vi "Wheel Angle (Ai).vi"(1 "Gamma ai":dbl, 2 "A":dbl) -> (0 "Ai":dbl)   [LabVIEW 2012]
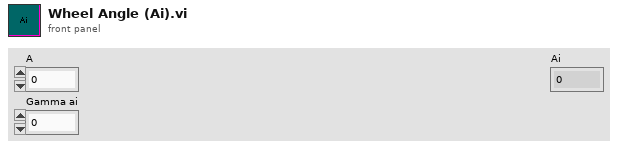
[diagram p1: front panel]
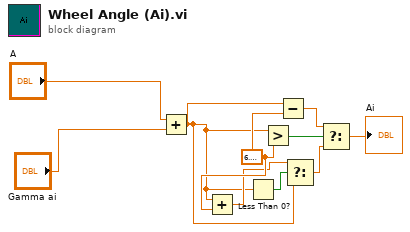
[diagram p0: block diagram]
diagram:
  w4 = 6.283185307179586
  n1 = Add(x="A", y="Gamma ai") -> (x+y=w2:dbl)
  n2 = Add(x=w2, y=w4) -> (x+y=w3:dbl)
  n3 = Less Than 0?(x=w2) -> (x < 0?=w5:bool)
  n4 = Greater?(x=w2, y=w4) -> (0:w8:bool)
  n5 = Subtract(x=w2, y=w4) -> (x-y=w7:dbl)
  n6 = Select(t=w3, s=w5, f=w2) -> (s? t:f=w6:dbl)
  n7 = Select(t=w7, s=w8, f=w6) -> (s? t:f=→"Ai":dbl)
